vi "ReadKeithley6485.vi"(8 "Error In":errorcluster, 11 "Keithley 6485 In":refnum<visa-resource-name>[](array[refnum])) -> (0 "Error Out":errorcluster, 2 "Data":dbl[](array[numeric]), 3 "Keithley 6485 Out":refnum<visa-resource-name>[](array[refnum]))   [LabVIEW 2012]
uses:
  libs/Keithley-6485/Keithley-6485.lvlib
  libs/LV-Utilities/LV-Utilities.lvlib
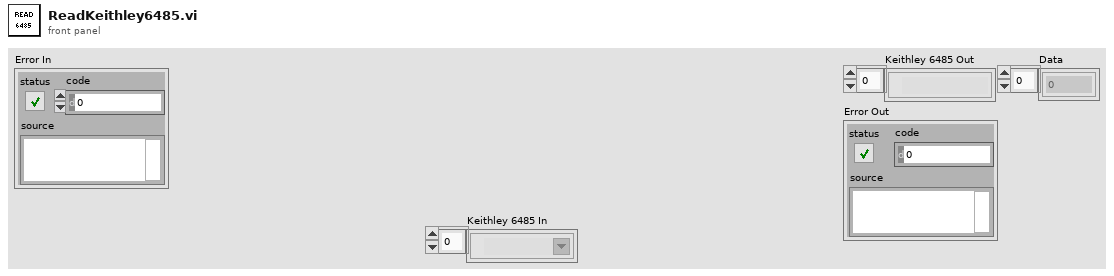
[diagram p1: front panel]
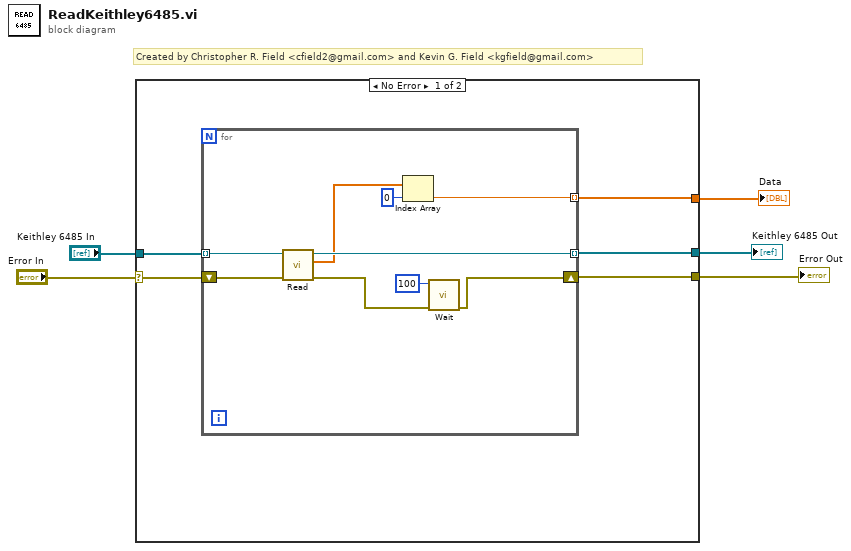
[diagram p0: block diagram]
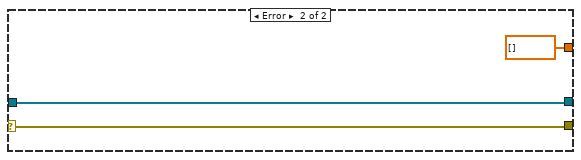
[diagram p2: hidden frame]
diagram:
  # "Created by Christopher R. Field <cfield2@gmail.com> and Kevin G. Field <kgfield@gmail.com>"
  n1 = case shown="No Error" "Error In" {
    selector: "Error In" -> [w7 w22]
    tunnel: "Keithley 6485 In" -> [w10 w21]
    tunnel: [w9 w21] -> w4
    tunnel: [w8 w22] -> w3
    tunnel: [w6 dbl[] []] -> w2
    frame No Error {
      n2 = for {
        tunnel: w10 -> [w18] mode=indexing
        shift-right: [w15] -> w8
        shift-left: w7 -> [w17]
        tunnel: [w19] -> w9 mode=indexing
        tunnel: [w11] -> w6 mode=indexing
        n3 = call "Read.vi"("Error In"=w17, "Keithley 6485 In"=w18) -> ("Error Out"=w16:errorcluster, "Values"=w13:dbl[], "Keithley 6485 Out"=w19:refnum<visa-resource-name>)  [unwired: 7 in]
        n4 = Index Array(array=w13, index=0) -> (element=w11:dbl)
        n5 = call "Wait.vi"("Error In"=w16, "Wait Time (msec)"=u32 100) -> ("Error Out"=w15:errorcluster)  [unwired: 9 in]
      }
    }
    frame Error {
    }
  }
  "Keithley 6485 Out" <- w4
  "Error Out" <- w3
  "Data" <- w2
